vi "Teleop.vi"(10 "Match Info":T1={"Autonomous Elapsed Seconds"=0.0, "TeleOp Elapsed Seconds"=0.0, "Disabled Elapsed Seconds"=0.0, "Visited Autonomous"=FALSE, "Visited TeleOp"=FALSE, "Visited Disabled"=FALSE, "Autonomous Settings"={"Autonomous Style"=enum."Independent", "VI Refnum"=refnum}}, 11 "Call Context":T2) -> ()   [LabVIEW 2015]
doc: "This VI is called for each TeleOp packet received from the DS where the robot is not disabled. It is often used to read from the joysticks and update I/O or to update setpoints for timed control loops. It should complete and return within 20 milliseconds or it may miss DS packets."
uses:
  <vilib>/Rock Robotics/Network Tables/NT Write Numeric Array.vi
  <vilib>/Rock Robotics/Network Tables/NT Read Boolean.vi
  <vilib>/Rock Robotics/Network Tables/NT Write Number.vi
  SlowMotion.vi
  <vilib>/Rock Robotics/Network Tables/NT Write Boolean.vi
  <vilib>/Rock Robotics/Network Tables/NT Write Boolean Array.vi
  <vilib>/Rock Robotics/Network Tables/NT Read Number.vi
  <vilib>/Rock Robotics/WPI/DriverStation/WPI_DriverStationMatch Info.ctl
  <vilib>/Rock Robotics/WPI/DriverStation/WPI_DriverStationDerivedRobotMode.ctl
panel:
  out "Sample Slider 0":dbl(slide) scale=0.0..5.0
  out "Sample Boolean 1":bool
  out "Sample Boolean 0":bool
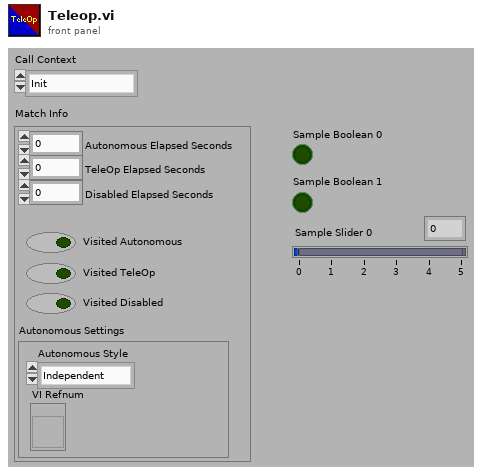
[diagram p1: front panel]
types:
  T1 = typedef "WPI_DriverStationMatch Info.ctl" = cluster{"Autonomous Elapsed Seconds":dbl, "TeleOp Elapsed Seconds":dbl, "Disabled Elapsed Seconds":dbl, "Visited Autonomous":bool, "Visited TeleOp":bool, "Visited Disabled":bool, "Autonomous Settings":cluster{"Autonomous Style":enum16{"Iterative", "Independent"}, "VI Refnum":refnum<vi>}}
  T2 = typedef "WPI_DriverStationDerivedRobotMode.ctl" = enum16{"Init", "Execute", "Stop"}
  T3 = typedef "WPI_JoystickDevRef.ctl" = cluster{"Device":T4}
  T4 = typedef "WPI_JoystickDeviceEnum.ctl" = enum16{"USB 0", "USB 1", "USB 2", "USB 3", "USB 4", "USB 5"}
  T5 = typedef "WPI_RobotDriveDevRef.ctl" = cluster{"DevStatus":errorcluster, "Motors[]":T6[], "Square Inputs":bool, "Max Output":dbl}
  T6 = typedef "WPI_MotorControlDeviceRef.ctl" = cluster{"DeviceStatus":errorcluster, "Type":T7, "PWM":cluster{"PWM Channel":T8, "DeadBand":T9}, "CAN":cluster{"Device Number":u8, "Control Mode":T10, "Semaphore":T11, "Max Vout":dbl, "TalonSRX Control Mode":T12}, "Invert":bool}
  T7 = typedef "WPI_MotorControlType.ctl" = enum16{"PWM", "CAN", "CANTalonSRX"}
  T8 = typedef "FPGA_DIOPWMChannel.ctl" = enum8{"PWM 0", "PWM 1", "PWM 2", "PWM 3", "PWM 4", "PWM 5", "PWM 6", "PWM 7", "PWM 8", "PWM 9", "PWM MXP 0", "PWM MXP 1", "PWM MXP 2", "PWM MXP 3", "PWM MXP 4", "PWM MXP 5", "PWM MXP 6", "PWM MXP 7", "PWM MXP 8", "PWM MXP 9", "Invalid"}
  T9 = typedef "WPI_PWMDeadband.ctl" = cluster{"Name":string, "maxPositivePwm":i32, "minPositivePwm":i32, "centerPwm":i32, "maxNegativePwm":i32, "minNegativePwm":i32, "angularRange":u16}
  T10 = typedef "WPI_CANJaguar_ControlMode.ctl" = enum8{"Percent VBus", "Current", "Speed", "Position", "Voltage"}
  T11 = typedef "Semaphore RefNum" = refnum<k1>
  T12 = typedef "WPI_CANTalonSRX_APIControlMode.ctl" = enum8{"Percent VBus", "Speed", "Position", "Slave", "Unchanged / Invalid", "Voltage Compensation", "Current", "Motion Profile"}
  T13 = typedef "WPI_SwitchDevRef.ctl" = cluster{"DevStatus":errorcluster, "DIO Channel":T14, "CntIndex":T15, "Normally Closed":bool}
  T14 = typedef "FPGA_DIOChannel.ctl" = enum8{"DIO 0", "DIO 1", "DIO 2", "DIO 3", "DIO 4", "DIO 5", "DIO 6", "DIO 7", "DIO 8", "DIO 9", "DIO MXP 0", "DIO MXP 1", "DIO MXP 2", "DIO MXP 3", "DIO MXP 4", "DIO MXP 5", "DIO MXP 6", "DIO MXP 7", "DIO MXP 8", "DIO MXP 9", "DIO MXP 10", "DIO MXP 11", "DIO MXP 12", "DIO MXP 13", "DIO MXP 14", "DIO MXP 15", "Invalid"}
  T15 = typedef "FPGA_CounterCtrSystemIndex.ctl" = enum8{"Ctr 0", "Ctr 1", "Ctr 2", "Ctr 3", "Ctr 4", "Ctr 5", "Ctr 6", "Ctr 7", "Invalid"}
  T16 = typedef "WPI_ServoDeviceRef.ctl" = cluster{"DeviceStatus":errorcluster, "PWM Channel":T8, "DeadBand":T9}
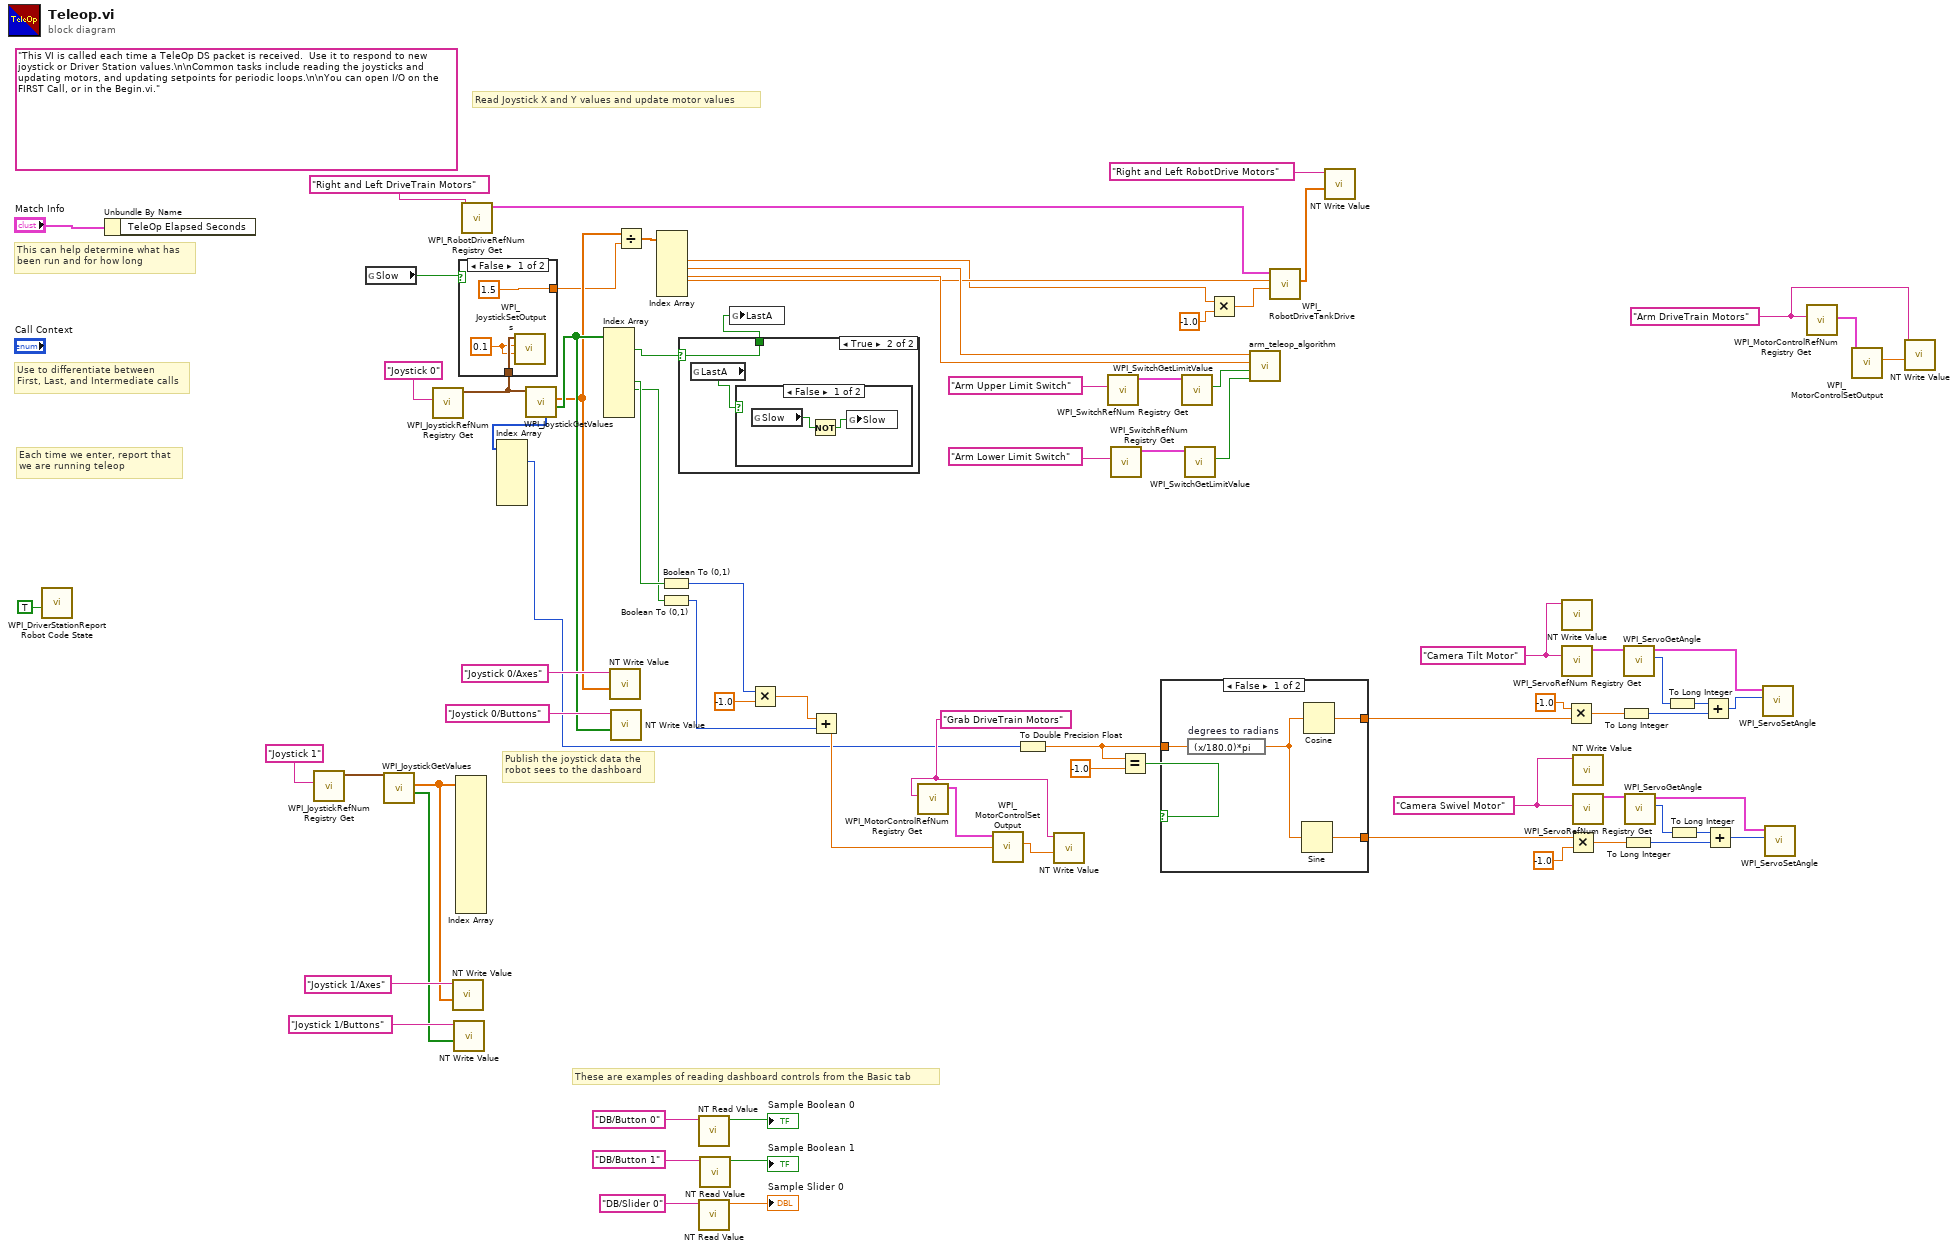
[diagram p0: block diagram]
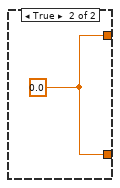
[diagram p2: hidden frame]
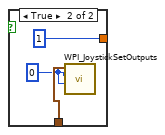
[diagram p3: hidden frame]
diagram:
  w23 = "Camera Swivel Motor" ("refnum name")
  w45 = "Camera Tilt Motor" ("refnum name")
  w53 = "Grab DriveTrain Motors" ("refnum name")
  w54 = "Arm DriveTrain Motors" ("refnum name")
  (unwired) "This VI is called each time a TeleOp DS packet is received.  Use it to respond to new joystick or Driver Station values.\n\nCommon tasks include reading the joysticks and updating motors, and updating setpoints for periodic loops.\n\nYou can open I/O on the FIRST Call, or in the Begin.vi."
  # "These are examples of reading dashboard controls from the Basic tab"
  # "Publish the joystick data the\nrobot sees to the dashboard"
  # "Each time we enter, report that\nwe are running teleop"
  # "Use to differentiate between\nFirst, Last, and Intermediate calls"
  # "This can help determine what has\nbeen run and for how long"
  # "Read Joystick X and Y values and update motor values"
  n1 = call <vilib>:"WPI_DriverStationReport Robot Code State.vi"("TeleOp"=TRUE ("Autonomous")) -> ()  [unwired: 10 in, 1 out]
  n2 = Unbundle By Name("Match Info") -> ()  [unwired: 1 out]
  n3 = call <vilib>:"WPI_JoystickRefNum Registry Get.vi"("refnum name"="Joystick 1") -> ("JoystickDevRef"=w9:T3)  [unwired: 1 in, 9 out]
  n4 = global read "SlowMotion.vi" "Slow"() -> (w48:bool)
  n5 = call <vilib>:"WPI_JoystickGetValues.vi"("JoystickDevRef"=w9) -> ("Buttons"=w5:bool[], "Axes"=w6:dbl[])  [unwired: 6 in, 3 out]
  n6 = call <vilib>:"WPI_JoystickRefNum Registry Get.vi"("refnum name"="Joystick 0") -> ("JoystickDevRef"=w46:T3)  [unwired: 1 in, 9 out]
  n7 = call-poly <vilib>:"NT Write Value.vi"("Numeric Array"=w6, "Name"="Joystick 1/Axes") -> ()  [unwired: 9 in, 1 out]
  n8 = call-poly <vilib>:"NT Write Value.vi"("Boolean Array"=w5, "Name"="Joystick 1/Buttons") -> ()  [unwired: 9 in, 1 out]
  n9 = Index Array(array=w6) -> ()  [unwired: 15 in, 15 out]
  n10 = case shown="False" w48 {
    tunnel: [1.5 1] -> w47
    tunnel: w46 -> [w83 w86]
    frame False {
      w82 = 0.1
      n11 = call <vilib>:"WPI_JoystickSetOutputs.vi"("Right Rumble"=w82, "Left Rumble"=w82, "JoystickDevRef"=w83) -> ()  [unwired: 7 in, 2 out]
    }
    frame True {
      w85 = 0
      n12 = call <vilib>:"WPI_JoystickSetOutputs.vi"("Right Rumble"=w85, "Left Rumble"=w85, "JoystickDevRef"=w86) -> ()  [unwired: 7 in, 2 out]
    }
  }
  n13 = call <vilib>:"WPI_RobotDriveRefNum Registry Get.vi"("refnum name"="Right and Left DriveTrain Motors") -> ("RobotDriveDevRef"=w68:T5)  [unwired: 1 in, 9 out]
  n14 = call <vilib>:"WPI_JoystickGetValues.vi"("JoystickDevRef"=w46) -> ("Buttons"=w65:bool[], "Axes"=w52:dbl[], "POVs"=w44:i16[])  [unwired: 6 in, 2 out]
  n15 = Index Array(array=w44) -> (element #1=w43:i16)  [unwired: 6 in, 5 out]
  n16 = Index Array(array=w65) -> (element #1=w50:bool, element #5=w60:bool, element #6=w58:bool)  [unwired: 9 in, 6 out]
  n17 = call-poly <vilib>:"NT Write Value.vi"("Numeric Array"=w52, "Name"="Joystick 0/Axes") -> ()  [unwired: 9 in, 1 out]
  n18 = call-poly <vilib>:"NT Write Value.vi"("Boolean Array"=w65, "Name"="Joystick 0/Buttons") -> ()  [unwired: 9 in, 1 out]
  n19 = Divide(x=w52, y=w47) -> (x/y=w51:dbl[])
  n20 = Index Array(array=w51) -> (element #2=w12:dbl, element #3=w22:dbl, element #4=w21:dbl, element #6=w13:dbl)  [unwired: 6 in, 2 out]
  n21 = Boolean To (0,1)(Boolean=w60) -> (0, 1=w59:i16)
  n22 = Boolean To (0,1)(Boolean=w58) -> (0, 1=w57:i16)
  n23 = case shown="True" w50 {
    selector: w50 -> [w88 w89]
    tunnel: [w88 w89] -> w49
    frame False {
    }
    frame True {
      n24 = global read "SlowMotion.vi" "LastA"() -> (w90:bool)
      n25 = case shown="False" w90 {
        frame False {
          n26 = global read "SlowMotion.vi" "Slow"() -> (w91:bool)
          n27 = Not(x=w91) -> (.not. x?=w92:bool)
          n28 = global write "SlowMotion.vi" "Slow"(w92) -> ()
        }
        frame True {
        }
      }
    }
  }
  n29 = call-poly <vilib>:"NT Read Value.vi"("Name"="DB/Button 0" ("refnum name")) -> ("Boolean"=→"Sample Boolean 0":bool)  [unwired: 9 in, 1 out]
  n30 = call-poly <vilib>:"NT Read Value.vi"("Name"="DB/Slider 0" ("refnum name")) -> ("Numeric"=→"Sample Slider 0":dbl)  [unwired: 9 in, 1 out]
  n31 = call-poly <vilib>:"NT Read Value.vi"("Name"="DB/Button 1" ("refnum name")) -> ("Boolean"=→"Sample Boolean 1":bool)  [unwired: 9 in, 1 out]
  n32 = global write "SlowMotion.vi" "LastA"(w49) -> ()
  n33 = Multiply(x=w59, y=-1.0) -> (x*y=w63:dbl)
  n34 = Add(x=w63, y=w57) -> (x+y=w62:dbl)
  n35 = call <vilib>:"WPI_MotorControlRefNum Registry Get.vi"("refnum name"=w53) -> ("MotorControlDevRef"=w61:T6)  [unwired: 9 in, 1 out]
  n36 = call <vilib>:"WPI_MotorControlSetOutput.vi"("Output"=w62, "MotorControlDevRef"=w61) -> ("Motor Output"=w55:dbl)  [unwired: 7 in, 2 out]
  n37 = To Double Precision Float(number=w43) -> (double precision float=w40:dbl)
  n38 = call-poly <vilib>:"NT Write Value.vi"("Numeric"=w55, "Name"=w53) -> ()  [unwired: 9 in, 1 out]
  n39 = call <vilib>:"WPI_SwitchRefNum Registry Get.vi"("refnum name"="Arm Upper Limit Switch") -> ("SwitchDevRef"=w19:T13)  [unwired: 9 in, 1 out]
  n40 = call <vilib>:"WPI_SwitchRefNum Registry Get.vi"("refnum name"="Arm Lower Limit Switch") -> ("SwitchDevRef"=w17:T13)  [unwired: 9 in, 1 out]
  n41 = Equal?(x=w40, y=-1.0) -> (x = y?=w41:bool)
  n42 = case shown="False" w41 {
    tunnel: [w95 w97] -> w4
    tunnel: [w96 w97] -> w39
    tunnel: w40 -> [w94 _]
    frame False {
      n43 = expression code="(x/180.0)*pi" "degrees to radians"(w94) -> (w93:dbl)
      n44 = Sine(x=w93) -> (sin(x)=w95:dbl)
      n45 = Cosine(x=w93) -> (cos(x)=w96:dbl)
    }
    frame True {
      w97 = 0.0
    }
  }
  n46 = call <vilib>:"WPI_SwitchGetLimitValue.vi"("SwitchDevRef"=w19) -> ("Switch Pressed"=w18:bool)  [unwired: 8 in, 2 out]
  n47 = call <vilib>:"WPI_SwitchGetLimitValue.vi"("SwitchDevRef"=w17) -> ("Switch Pressed"=w15:bool)  [unwired: 8 in, 2 out]
  n48 = Multiply(x=w12, y=-1.0) -> (x*y=w11:dbl)
  n49 = call "arm_teleop_algorithm.vi"("Lower Limit Reached"=w15, "Upper Limit Reached"=w18, "Arm Move Down"=w21, "Arm Move Up"=w22) -> ("x+y"=w2:dbl)  [unwired: 7 in]
  n50 = call <vilib>:"WPI_RobotDriveTankDrive.vi"("Right axis value"=w11, "Left axis value"=w13, "RobotDriveDevRef"=w68) -> ("Motor Values"=w67:dbl[])  [unwired: 6 in, 2 out]
  n51 = call-poly <vilib>:"NT Write Value.vi"("Numeric Array"=w67, "Name"="Right and Left RobotDrive Motors") -> ()  [unwired: 9 in, 1 out]
  n52 = call-poly <vilib>:"NT Write Value.vi"("Name"=w45) -> ()  [unwired: 10 in, 1 out]
  n53 = call <vilib>:"WPI_ServoRefNum Registry Get.vi"("refnum name"=w45) -> ("ServoDeviceRef"=w36:T16)  [unwired: 9 in, 1 out]
  n54 = Multiply(x=-1.0, y=w39) -> (x*y=w37:dbl)
  n55 = Multiply(x=w4, y=-1.0 ("x")) -> (x*y=w24:dbl)
  n56 = call-poly <vilib>:"NT Write Value.vi"("Name"=w23) -> ()  [unwired: 10 in, 1 out]
  n57 = call <vilib>:"WPI_ServoRefNum Registry Get.vi"("refnum name"=w23) -> ("ServoDeviceRef"=w25:T16)  [unwired: 9 in, 1 out]
  n58 = To Long Integer(number=w37) -> (32bit integer=w34:i32)
  n59 = To Long Integer(number=w24) -> (32bit integer=w27:i32)
  n60 = call <vilib>:"WPI_ServoGetAngle.vi"("ServoDeviceRef"=w36) -> ("ServoDeviceRef"=w33:T16, "Angle"=w35:u16)  [unwired: 7 in, 1 out]
  n61 = call <vilib>:"WPI_ServoGetAngle.vi"("ServoDeviceRef"=w25) -> ("ServoDeviceRef"=w28:T16, "Angle"=w26:u16)  [unwired: 7 in, 1 out]
  n62 = To Long Integer(number=w35) -> (32bit integer=w32:i32)
  n63 = To Long Integer(number=w26) -> (32bit integer=w29:i32)
  n64 = Add(x=w32, y=w34) -> (x+y=w31:i32)
  n65 = Add(x=w29, y=w27) -> (x+y=w30:i32)
  n66 = call <vilib>:"WPI_ServoSetAngle.vi"("Angle"=w31, "ServoDeviceRef"=w33) -> ()  [unwired: 8 in, 2 out]
  n67 = call <vilib>:"WPI_ServoSetAngle.vi"("Angle"=w30, "ServoDeviceRef"=w28) -> ()  [unwired: 8 in, 2 out]
  n68 = call <vilib>:"WPI_MotorControlRefNum Registry Get.vi"("refnum name"=w54) -> ("MotorControlDevRef"=w66:T6)  [unwired: 9 in, 1 out]
  n69 = call <vilib>:"WPI_MotorControlSetOutput.vi"("MotorControlDevRef"=w66) -> ("Motor Output"=w56:dbl, "Output"=w1:dbl)  [unwired: 7 in, 2 out]
  n70 = call-poly <vilib>:"NT Write Value.vi"("Numeric"=w56, "Name"=w54) -> ()  [unwired: 9 in, 1 out]
